vi "GetCCMValue.vi"(0 "TT1 F":dbl, 5 "CMM":dbl[][](array[numeric])) -> (4 "WBLimit":dbl, 6 "PBLimit":dbl, 8 "EGTLimit":dbl)   [LabVIEW 2018, in "Controller (Host).lvlib"]
uses:
  Controller (Host).lvlib
panel:
  # "TT1C"
  # "TTI F"
  # "WBCOR"
  # "PBCOR"
  # "EGTCOR F"
  # "EGTCOR C"
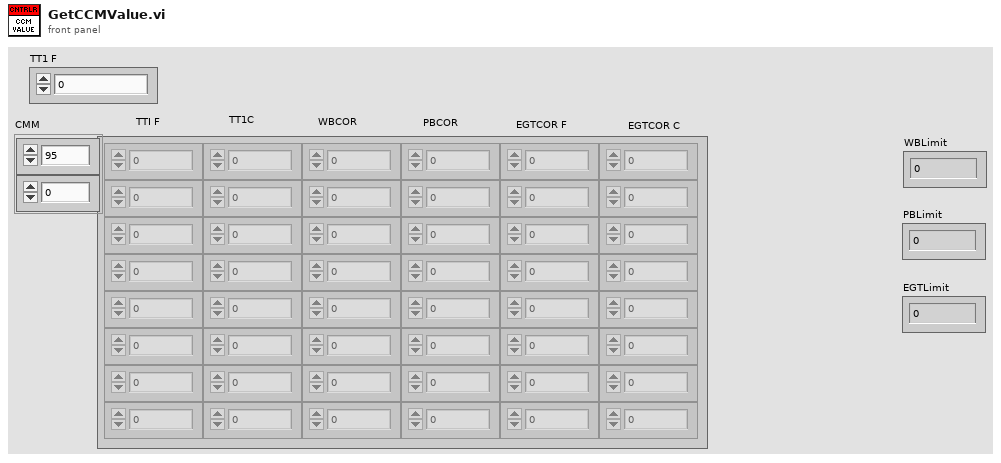
[diagram p1: front panel]
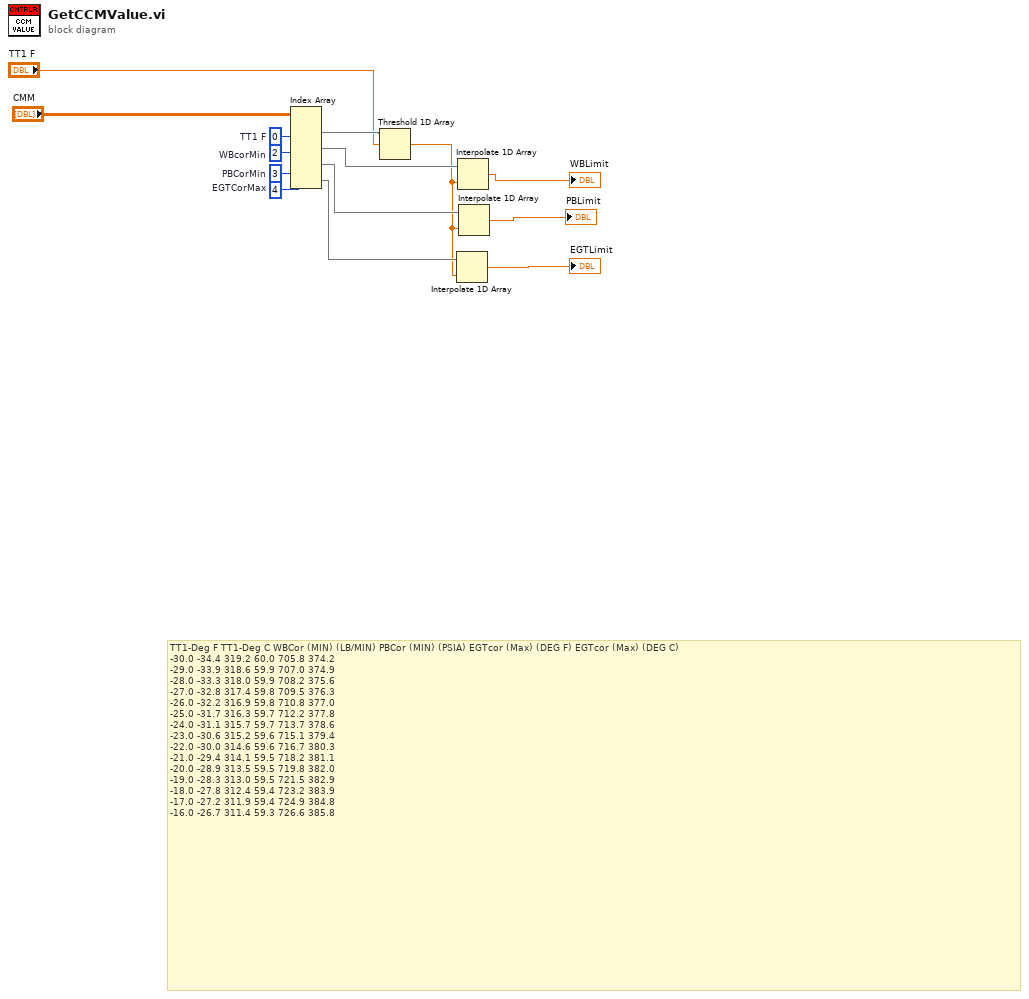
[diagram p0: block diagram]
diagram:
  w11 = 4  # EGTCorMax
  w12 = 3  # PBCorMin
  w13 = 2  # WBcorMin
  w14 = 0  # TT1 F
  # "TT1-Deg F\tTT1-Deg C\tWBCor (MIN) (LB/MIN)\tPBCor (MIN) (PSIA)\tEGTcor (Max) (DEG F)\tEGTcor (Max) (DEG C)\n-30.0\t-34.4\t319.2\t60.0\t705.8\t374.2\n-29.0\t-33.9\t318.6\t59.9\t707.0\t374.9\n-28.0\t-33.3\t318.0\t59.9\t708.2\t375.6\n-27.0\t-32.8\t317.4\t59.8\t709.5\t376.3\n-26.0\t-32.2\t316.9\t59.8\t710.8\t377.0\n-25.0\t-31.7\t316.3\t59.7\t712.2\t377.8\n-24.0\t-31.1\t315.7\t59.7\t713.7\t378.6\n-23.0\t-30.6\t315.2\t59.6\t715.1\t379.4\n-22.0\t-30.0\t314.6\t59.6\t716.7\t380.3\n-21.0\t-29.4\t314.1\t59.5\t718.2\t381.1\n-20.0\t-28.9\t313.5\t59.5\t719.8\t382.0\n-19.0\t-28.3\t313.0\t59.5\t721.5\t382.9\n-18.0\t-27.8\t312.4\t59.4\t723.2\t383.9\n-17.0\t-27.2\t311.9\t59.4\t724.9\t384.8\n-16.0\t-26.7\t311.4\t59.3\t726.6\t385.8"
  n1 = Index Array(array="CMM", index (col) #1=w14, index (col) #2=w13, index (col) #3=w12, index (col) #4=w11) -> (element #1=w10:dbl[], element #2=w9:dbl[], element #3=w7:dbl[], element #4=w5:dbl[])  [unwired: 4 in]
  n2 = Threshold 1D Array(2:"TT1 F", 3:w10) -> (0:w4:dbl)  [unwired: 1 in]
  n3 = Interpolate 1D Array(1:w4, 2:w5) -> (0:→"EGTLimit":dbl)
  n4 = Interpolate 1D Array(1:w4, 2:w9) -> (0:→"WBLimit":dbl)
  n5 = Interpolate 1D Array(1:w4, 2:w7) -> (0:→"PBLimit":dbl)
